vi "Generate Random Bytes.vi"(8 "error in (no error)":errorcluster, 11 "byte count":i32) -> (0 "error out":errorcluster, 3 "random data (U8)":u8[](array[numeric]))   [LabVIEW 2021, in "dotNET Crypto RNG.lvlib"]
doc: "Generate random bytes of data using a cryptographically secure algorithm."
uses:
  dotNET Crypto RNG.lvlib
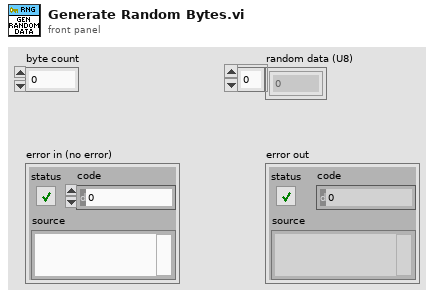
[diagram p1: front panel]
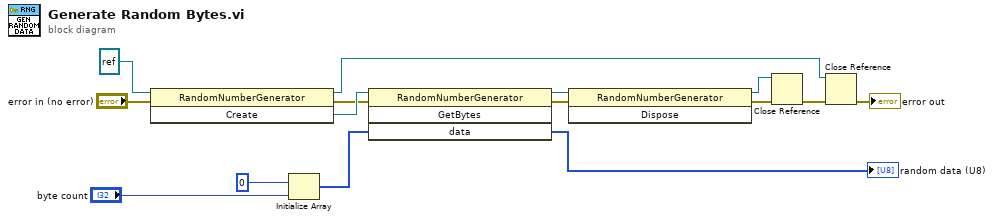
[diagram p0: block diagram]
diagram:
  n1 = invoke class="RandomNumberGenerator" method="Create"(reference=refnum<k24> refnum, error in="error in (no error)") -> (reference out=w2:refnum<k24>, error out=w6:errorcluster, "Create"=w7:refnum<k24>)  [unwired: 1 in]
  n2 = Initialize Array(u8 0, "byte count") -> (w10:u8[])
  n3 = invoke class="RandomNumberGenerator" method="GetBytes"(reference=w7, error in=w6, "data"=w10) -> (reference out=w15:refnum<k24>, error out=w12:errorcluster, "data"=→"random data (U8)":u8[])  [unwired: 1 in, 1 out]
  n4 = invoke class="RandomNumberGenerator" method="Dispose"(reference=w15, error in=w12) -> (reference out=w14:refnum<k24>, error out=w13:errorcluster)  [unwired: 1 in, 1 out]
  n5 = Close Reference(reference=w14, error in (no error)=w13) -> (error out=w4:errorcluster)
  n6 = Close Reference(reference=w2, error in (no error)=w4) -> (error out=→"error out":errorcluster)
